vi "Create Table.vi"(8 "error in (no error)":errorcluster, 11 "MySQL in":refnum<class "MySQL.lvclass">) -> (0 "error out":errorcluster, 3 "MySQL out":refnum<class "MySQL.lvclass">)   [LabVIEW 2016, in "Database.lvlib" / "MySQL.lvclass"]
uses:
  MySQL.lvclass
  DB/DB.lvclass
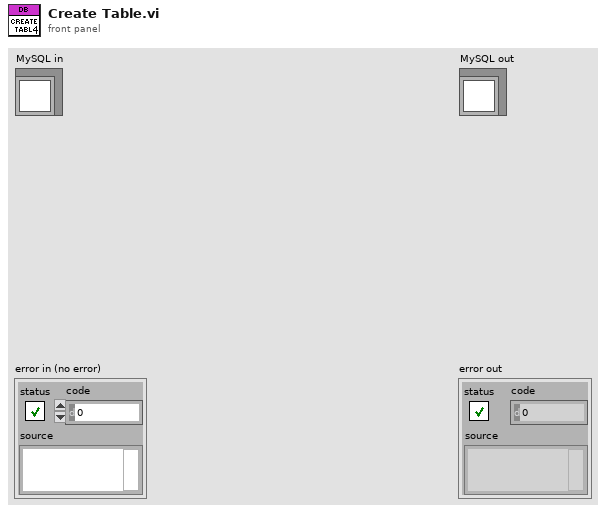
[diagram p1: front panel]
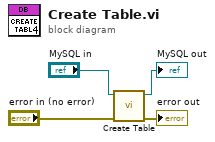
[diagram p0: block diagram]
diagram:
  n1 = call-parent "Create Table.vi"("error in (no error)"="error in (no error)", "DB in"="MySQL in") -> ("error out"=→"error out":errorcluster, "DB out"=→"MySQL out":refnum<class "MySQL.lvclass">)  [unwired: 8 in]
